vi "detect controller.vi"(10 "Device Model":enum16{"cRIO-9068"}(ring)) -> (0 "error out":errorcluster, 2 "passed?":bool)   [LabVIEW 2013, in "SMI Tests.lvlib"]
uses:
  SMI Tests.lvlib
  classes/SysCfg Device/SysCfg Device.lvclass
  classes/Controller/Controller.lvclass
  <vilib>/utf/common/utf_test_result.ctl
  <vilib>/utf/NI_UnitTestFramework.lvlib
  <vilib>/utf/common/utf_vi_tag.ctl
  <vilib>/utf/common/utf_test_comparison_operators.ctl
  <vilib>/utf/common/utf_test_result_failure.ctl
  <vilib>/utf/common/utf_test_result_troll.ctl
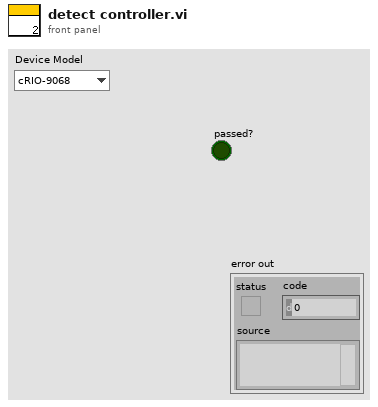
[diagram p1: front panel]
types:
  T1 = typedef "SMI.lvlib/Controller.lvclass/controller information.ctl" = cluster{"system session":refnum<data-value>, "system hardware ref":refnum<data-value>, "vendor name":string, "product name":string, "product ID":u16, "serial number":string, "device information":T2, "primary network adapter":T3, "secondary network adapters":T3[]}
  T2 = typedef "SMI.lvlib/Controller.lvclass/device information.ctl" = cluster{"resource":string, "device class":string, "system start time":timestamp, "current time":timestamp, "time zone":string, "firmware revision":string, "image title":string, "image version":string, "system status":string}
  T3 = typedef "SMI.lvlib/Controller.lvclass/network adapter settings.ctl" = cluster{"IP address":string, "MAC address":string, "IP address request mode":u32, "subnet mask":string, "gateway":string, "DNS server":string, "adapter mode":u32, "adapter type":u32}
  T4 = typedef "NI_UnitTestFramework.lvlib/utf_test_result_troll.ctl" = cluster{"time elapsed [ms]":u32, "result (test)":T5, "result (parameters)":T6[]}
  T5 = typedef "NI_UnitTestFramework.lvlib/utf_test_result.ctl" = enum16{"Passed", "Failed", "Error", "Skipped", "Not Processed"}
  T6 = typedef "NI_UnitTestFramework.lvlib/utf_test_result_failure.ctl" = cluster{"result":T5, "error message":string, "parameter name":string, "parameter value":variant, "parameters":variant[], "comparison":T7, "requirement ID":string, "VI":T8, "Used Vector Name":string}
  T7 = typedef "NI_UnitTestFramework.lvlib/utf_test_comparison_operators.ctl" = enum16{"=", "!=", ">", ">=", "<", "<=", "range", "symmetric tolerance", "asymmetric tolerance", "string contains", "string not contain", "array size", "string length", "array range", "by element", "array range (limit array)", "user-defined", "array contains", "array not contain", "vector length", "= (elm)", "!= (elm)", "= (case insensitive)", "!= (case insensitive)"}
  T8 = typedef "NI_UnitTestFramework.lvlib/utf_vi_tag.ctl" = enum16{"Setup VI", "VI under Test", "Teardown VI"}
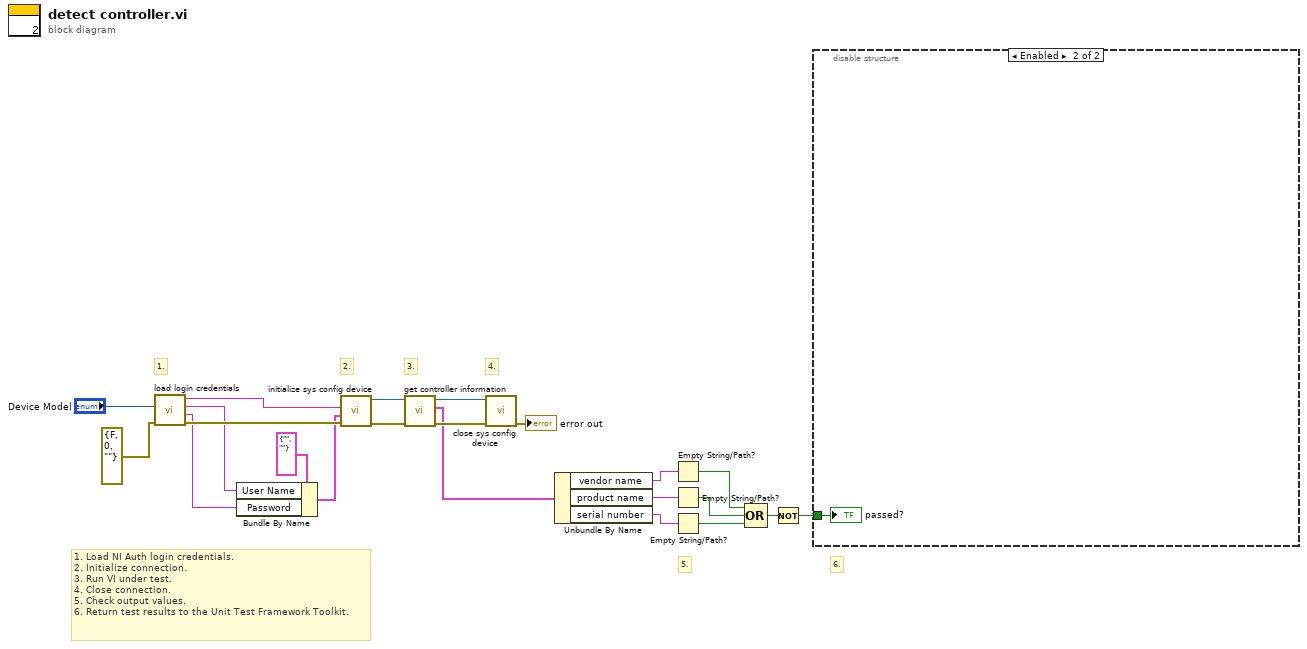
[diagram p0: block diagram]
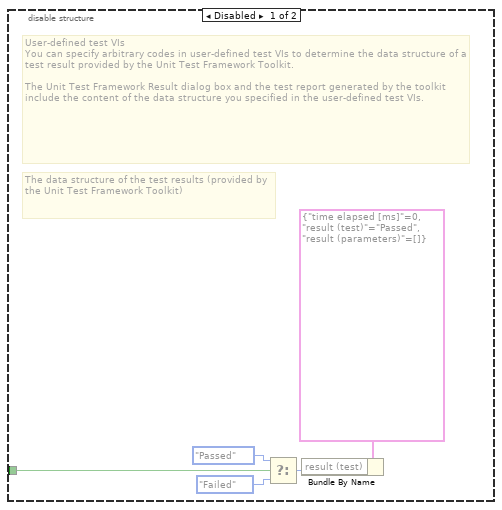
[diagram p2: hidden frame]
diagram:
  # "6."
  # "4."
  # "1. Load NI Auth login credentials.\n2. Initialize connection.\n3. Run VI under test.\n4. Close connection.\n5. Check output values.\n6. Return test results to the Unit Test Framework Toolkit."
  # "2."
  # "1."
  # "3."
  # "5."
  n1 = call "load login credentials.vi"("error in"=errorcluster {"status"=FALSE, "code"=0, "source"=""}, "Device Model"="Device Model") -> ("error out"=w22:errorcluster, "Password"=w17:string, "Username"=w18:string, "IP Address"=w16:string)  [unwired: 6 in]
  n2 = Bundle By Name(cluster=cluster{"User Name":string, "Password":string} {"User Name"="", "Password"=""} ("NI Auth (Unconfigured)"), "User Name"=w18, "Password"=w17) -> (w15:cluster{"User Name":string, "Password":string})
  n3 = call "initialize sys config device.vi"("error in"=w22, "login"=w15, "IP address (localhost)"=w16) -> ("error out"=w21:errorcluster, "Controller out"=w14:refnum<class "Controller.lvclass">)  [unwired: 7 in]
  n4 = call "get controller information.vi"("error in"=w21, "Controller in"=w14) -> ("error out"=w20:errorcluster, "controller information"=w11:T1, "Controller out"=w13:refnum<class "Controller.lvclass">)  [unwired: 7 in]
  n5 = call "close sys config device.vi"("error in"=w20, "Controller in"=w13) -> ("error out"=→"error out":errorcluster)  [unwired: 9 in]
  n6 = Unbundle By Name(w11) -> ("vendor name"=w8:string, "product name"=w7:string, "serial number"=w10:string)
  n7 = Empty String/Path?(string/path=w8) -> (empty?=w6:bool)
  n8 = Empty String/Path?(string/path=w7) -> (empty?=w5:bool)
  n9 = Empty String/Path?(string/path=w10) -> (empty?=w4:bool)
  n10 = Compound Arithmetic op=OR(w6, w5, w4) -> (w3:bool)
  n11 = Not(x=w3) -> (.not. x?=w2:bool)
  n12 = disable-structure shown="Enabled" {
    disable-tunnel: w2 -> [w23 w28]
    frame Disabled {
      # "User-defined test VIs\nYou can specify arbitrary codes in user-defined test VIs to determine the data structure of a test result provided by the Unit Test Framework Toolkit.\n\nThe Unit Test Framework Result dialog box and the test report generated by the toolkit include the content of the data structure you specified in the user-defined test VIs."
      # "The data structure of the test results (provided by the Unit Test Framework Toolkit)"
      n13 = Select(t=utf_test_result."Passed" ("Result (Test)"), s=w23, f=utf_test_result."Failed" ("Result (Test)")) -> (s? t:f=w27:T5)
      n14 = Bundle By Name(cluster=T4 {"time elapsed [ms]"=0, "result (test)"=enum."Passed", "result (parameters)"=[]} ("Constant"), "result (test)"=w27) -> ()  [unwired: 1 out]
    }
    frame Enabled {
      "passed?" <- w28
    }
  }
